vi "动态界面.vi"() -> ()   [LabVIEW 2018]
panel:
  in  "帮助信息":bool
  in  "stop":bool
  in  "设计思想":bool
  in  "采集":bool
  in  "发射":bool
  # "地学虚拟仪器电法勘测发射采集一体化系统"
  # "小组成员\n张所鑫\n李浚源\n张海萌"
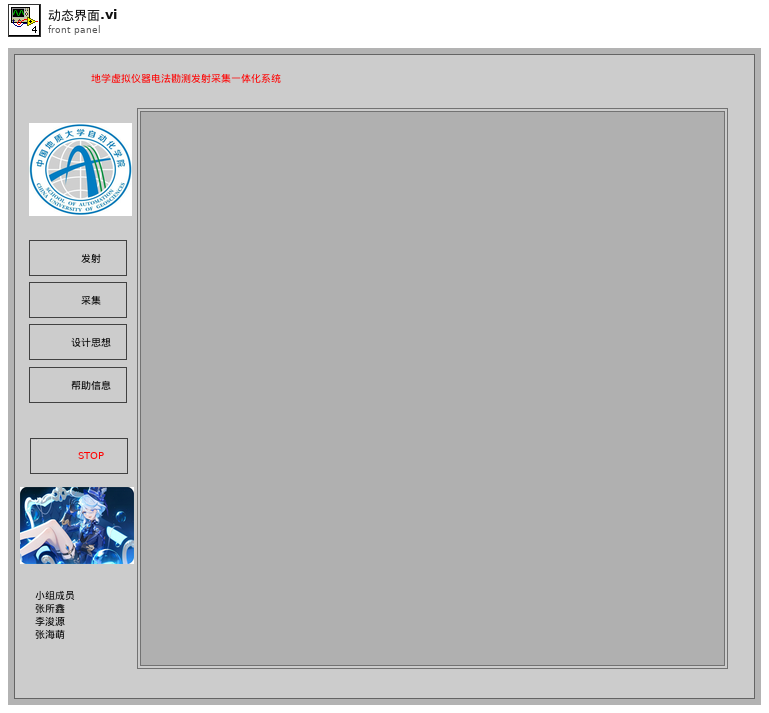
[diagram p1: front panel]
types:
  T1 = enum32{"Bad", "Idle", "Run top level", "Running"}
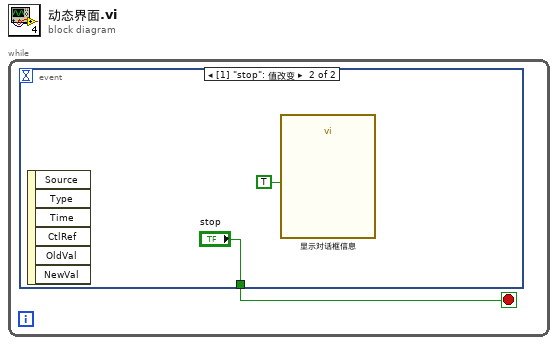
[diagram p0: block diagram]
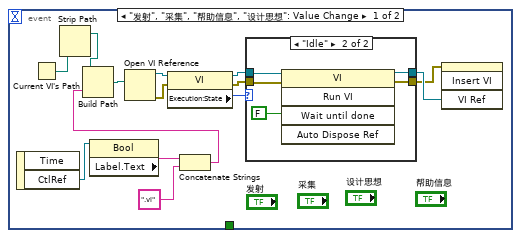
[diagram p2: hidden frame]
diagram:
  n1 = while {
    stop <- w1 stop-if-true
    n2 = event shown="[1] \"stop\": 值改变" {
      selector: _ -> [_ _]
      dyn-events: _ -> [_ _]
      timeout: _ -> [_ _]
      tunnel: [_ "stop"] -> w1
      event "发射", "采集", "帮助信息", "设计思想": Value Change {
        n3 = event-data() -> ("CtlRef"=w15:refnum<vi>)  [unwired: 2 out]
        n4 = Current VI's Path() -> (path=w3:path)
        n5 = Strip Path(path=w3) -> (stripped path=w2:path)  [unwired: 1 out]
        n6 = property class="Bool"(reference=w15) -> ("Label.Text"=w14:string)  [unwired: 1 in, 2 out]
        n7 = Concatenate Strings(w14, ".vi" ("string")) -> (w13:string)
        n8 = Build Path(base path=w2, name or relative path=w13) -> (appended path=w12:path)
        n9 = Open VI Reference(vi path=w12) -> (vi reference=w7:refnum<vi>, error out=w6:errorcluster)  [unwired: 1 in, 4 out]
        n10 = property on="Status" class="VI"(reference=w7, error in=w6) -> (reference out=w8:refnum<vi>, error out=w9:errorcluster, "Execution:State"=w10:T1)
        n11 = case shown="\"Idle\"" w10 {
          tunnel: [w17 w22] -> w5
          tunnel: [w16 w21] -> w4
          tunnel: w8 -> [w17 w20]
          tunnel: w9 -> [w16 w19]
          frame Default {
          }
          frame "Idle" {
            n12 = invoke class="VI" method="Run VI"(reference=w20, error in=w19, "Wait until done"=FALSE ("Wait Until Done")) -> (reference out=w22:refnum<vi>, error out=w21:errorcluster)  [unwired: 2 in, 3 out]
          }
        }
        n13 = invoke class="SubPanel" method="Insert VI"(error in=w4, "VI Ref"=w5) -> ()  [unwired: 2 in, 4 out]
      }
      event "stop": Value Change {
        n14 = event-data() -> ()  [unwired: 7 out]
        n15 = call "显示对话框信息"("Enable"=TRUE) -> ()  [unwired: 9 in, 2 out]
      }
    }
  }
